vi "ARINC word test.vi"(11 "ARINC word in":T1 {"ARINC word" format="%032b"}) -> (3 "ARINC word out":T1 {"ARINC word" format="%032b"})   [LabVIEW 2012]
uses:
  RT/Typdefs/ARINC word cluster.ctl
  RT/Typdefs/ARINC word.ctl
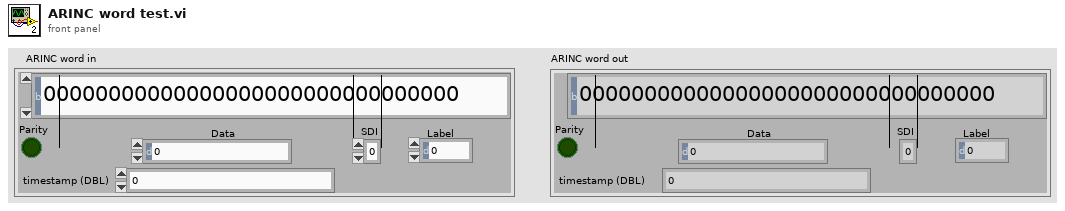
[diagram p1: front panel]
types:
  T1 = typedef "ARINC word cluster.ctl" = cluster{"ARINC word":T2, "Label":u8, "SDI":u8, "Data":u32, "Parity":bool, "timestamp (DBL)":dbl}
  T2 = typedef "ARINC word.ctl" = u32
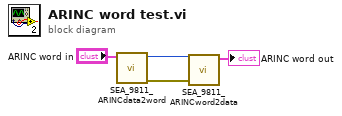
[diagram p0: block diagram]
diagram:
  n1 = call "SEA_9811_ARINCdata2word.vi"("ARINC word in"="ARINC word in") -> ("error out"=w3:errorcluster, "ARINC word out"=w4:T2)  [unwired: 9 in]
  n2 = call "SEA_9811_ARINCword2data.vi"("error in (no error)"=w3, "ARINC word in"=w4) -> ("ARINC word out"=→"ARINC word out":T1)  [unwired: 8 in, 1 out]
